vi "Read Array of Cells.vi"(8 "error in (no error)":errorcluster, 11 "Schedule in":refnum<class "Schedule.lvclass">) -> (0 "error out":errorcluster, 2 "RUNs":refnum<class "Schedule Cell.lvclass">[](array[class]), 3 "Schedule out":refnum<class "Schedule.lvclass">)   [LabVIEW 2020, in "TALOS.lvlib" / "Run Utilities.lvlib" / "Schedule.lvclass"]
uses:
  Schedule.lvclass
  Cell/Schedule Cell.lvclass
  Schedule.lvclass/Schedule.ctl
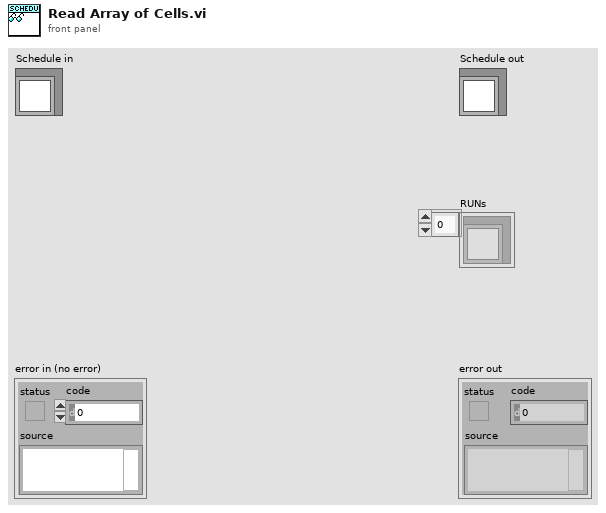
[diagram p1: front panel]
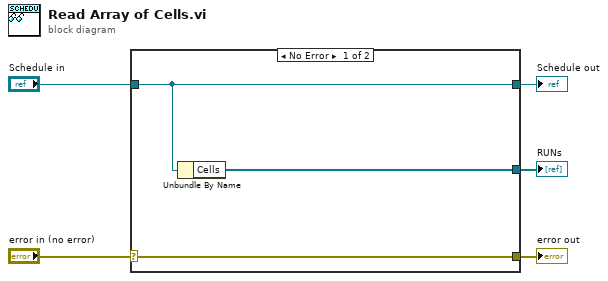
[diagram p0: block diagram]
diagram:
  n1 = case shown="No Error" "error in (no error)" {
    selector: "error in (no error)" -> [w8 w9]
    tunnel: [w8 w9] -> w4
    tunnel: [w7 w10] -> w2
    tunnel: "Schedule in" -> [w7 w10]
    tunnel: [w6 _] -> w1
    frame No Error {
      n2 = Unbundle By Name(w7) -> ("Cells"=w6:refnum<class "Schedule Cell.lvclass">[])
    }
    frame Error {
    }
  }
  "error out" <- w4
  "Schedule out" <- w2
  "RUNs" <- w1
